vi "intensity graph.vi"() -> ()   [LabVIEW 2012]
panel:
  out "Intensity Graph":dbl[][](graph)
  in  "Array":dbl[][](array[numeric])
  in  "stop":bool
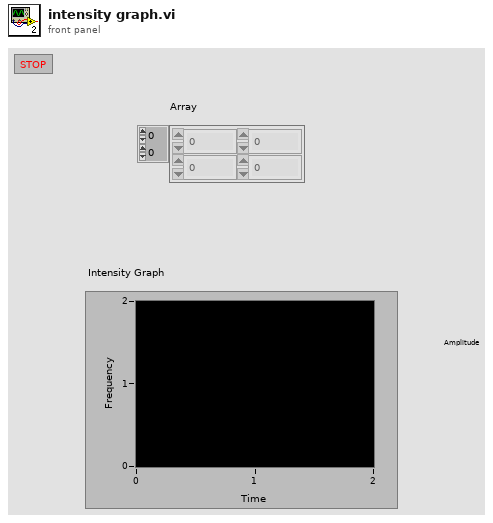
[diagram p1: front panel]
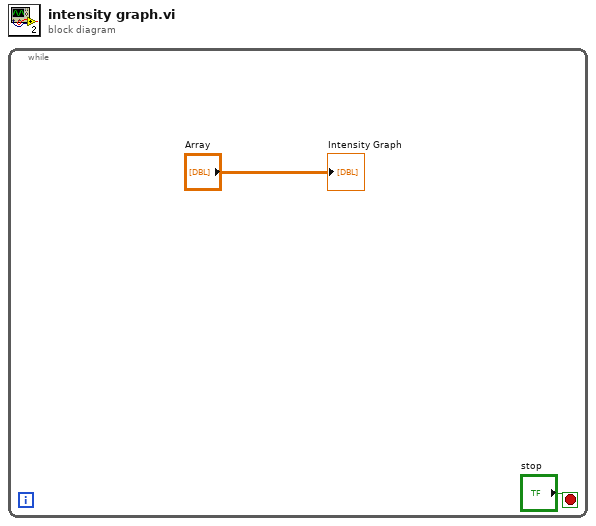
[diagram p0: block diagram]
diagram:
  n1 = while {
    stop <- "stop" stop-if-true
    "Intensity Graph" <- "Array"
  }
